vi "ZaberRenumber.vi"(6 "max speed (mm/s)":dbl, 8 "resolution":dbl, 11 "VISA Refnum in":refnum<visa-resource-name>) -> (0 "error out":errorcluster, 1 "Device 1":string, 2 "Device 0":string, 3 "VISA Refnum out":refnum<visa-resource-name>, 4 "X-axis Device":string, 5 "Y-axis Device":string)   [LabVIEW 2011]
uses:
  Zaber/Zaber A Series.lvlib
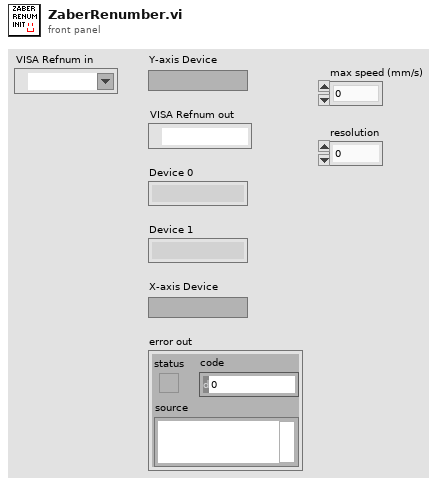
[diagram p1: front panel]
types:
  T1 = cluster{"Device":string, "Axis":string, "Reply Flag":string, "Status":string, "Warning Flags":string, "Data":string}[]
  T2 = cluster{"Device":string, "Axis":string, "Reply Flag":string, "Status":string, "Warning Flags":string, "Data":string}
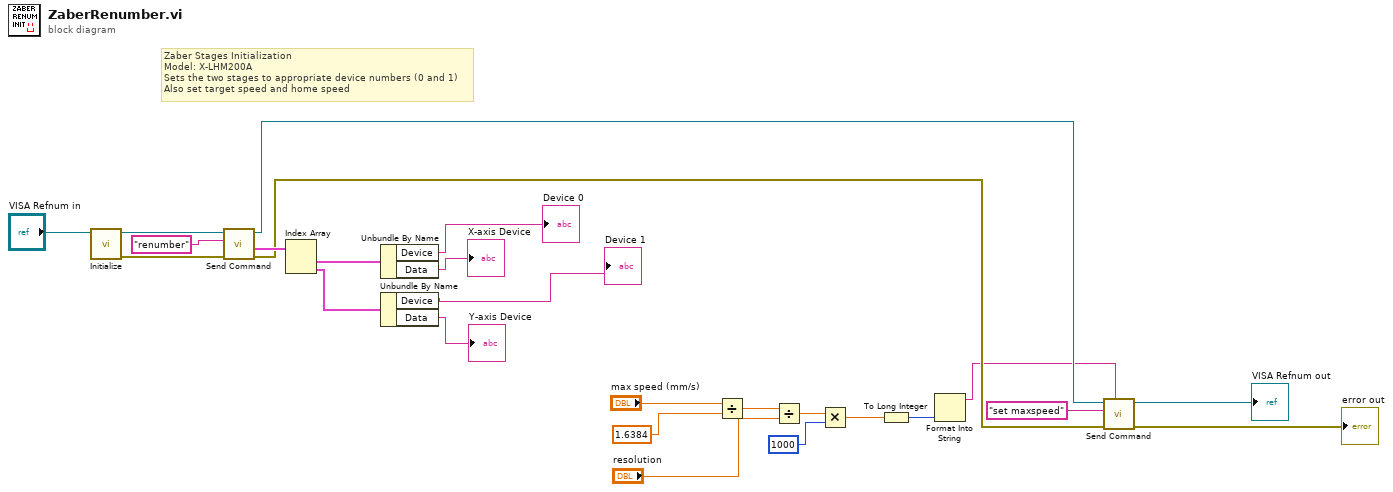
[diagram p0: block diagram]
diagram:
  # "Zaber Stages Initialization\nModel: X-LHM200A\nSets the two stages to appropriate device numbers (0 and 1)\nAlso set target speed and home speed"
  n1 = call "Initialize.vi"("VISA resource name"="VISA Refnum in") -> ("error out"=w17:errorcluster, "VISA resource name out"=w16:refnum<visa-resource-name>)  [unwired: 9 in]
  n2 = call "Send Command.vi"("error in (no error)"=w17, "Command"="renumber", "VISA resource name"=w16) -> ("error out"=w4:errorcluster, "Response Bundle Array"=w19:T1, "VISA resource name out"=w5:refnum<visa-resource-name>)  [unwired: 4 in, 2 out]
  n3 = Index Array(array=w19) -> (element #1=w20:T2, element #2=w21:T2)  [unwired: 2 in]
  n4 = Unbundle By Name(w20) -> ("Device"=→"Device 0":string, "Data"=→"X-axis Device":string)
  n5 = Unbundle By Name(w21) -> ("Device"=→"Device 1":string, "Data"=→"Y-axis Device":string)
  n6 = Divide(x="max speed (mm/s)", y=1.6384) -> (x/y=w9:dbl)
  n7 = Divide(x=w9, y="resolution") -> (x/y=w8:dbl)
  n8 = Multiply(x=w8, y=1000) -> (x*y=w6:dbl)
  n9 = To Long Integer(number=w6) -> (32bit integer=w11:i32)
  n10 = Format Into String(w11) -> (resulting string=w3:string)  [unwired: 3 in, 1 out]
  n11 = call "Send Command.vi"("Data"=w3, "error in (no error)"=w4, "Command"="set maxspeed", "VISA resource name"=w5) -> ("error out"=→"error out":errorcluster, "VISA resource name out"=→"VISA Refnum out":refnum<visa-resource-name>)  [unwired: 3 in, 3 out]
